vi "Field Add Test Step Fields to Table.vi"(8 "error in (no error)":errorcluster, 10 "Fields":T1[](array[typedef]), 11 "Connection Refnum":T4) -> (0 "error out":errorcluster, 3 "Connection Refnum":T4)   [LabVIEW 2011]
uses:
  SI.LIB/ODBC/SQL Controls/Connection Refnum.ctl
  Field Record.ctl
  Field DataTypes.ctl
  Field NextItem.ctl
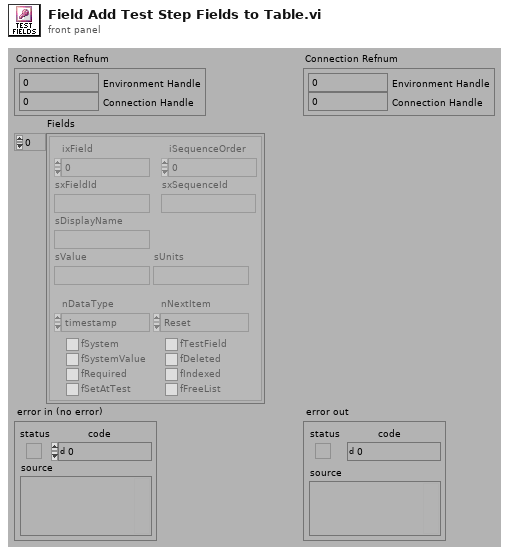
[diagram p1: front panel]
types:
  T1 = typedef "Field Record.ctl" = cluster{"ixField":i32, "iSequenceOrder":i32, "sxFieldId":string, "sxSequenceId":string, "sDisplayName":string, "sValue":string, "sUnits":string, "nDataType":T2, "nNextItem":T3, "fSystem":bool, "fSystemValue":bool, "fRequired":bool, "fSetAtTest":bool, "fTestField":bool, "fDeleted":bool, "fIndexed":bool, "fFreeList":bool}
  T2 = typedef "Field DataTypes.ctl" = enum32{"text", "numeric", "list", "timestamp", "boolean"}
  T3 = typedef "Field NextItem.ctl" = enum32{"Reset", "Retain", "Auto-Increment"}
  T4 = typedef "Connection Refnum.ctl" = cluster{"Environment Handle":i32, "Connection Handle":i32}
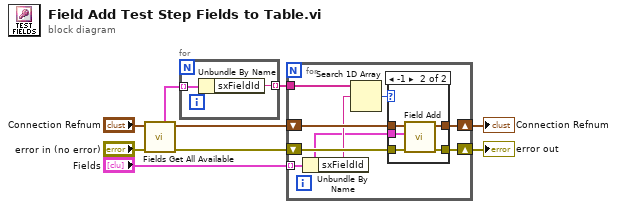
[diagram p0: block diagram]
diagram:
  n1 = call "Fields Get All Available.vi"("error in (no error)"="error in (no error)", "Connection Refnum"="Connection Refnum") -> ("error out"=w4:errorcluster, "Connection Refnum"=w5:T4, "Test Fields"=w1:T1[])  [unwired: 3 in, 4 out]
  n2 = for {
    tunnel: w1 -> [w11] mode=indexing
    tunnel: [w10] -> w2 mode=indexing
    n3 = Unbundle By Name(w11) -> ("sxFieldId"=w10:string)
  }
  n4 = for {
    shift-right: [w19] -> w8
    shift-left: w5 -> [w16]
    shift-right: [w18] -> w6
    shift-left: w4 -> [w17]
    tunnel: "Fields" -> [w12] mode=indexing
    tunnel: w2 -> [w15]
    n5 = Unbundle By Name(w12) -> ("sxFieldId"=w14:string)
    n6 = Search 1D Array(1D array=w15, element=w14) -> (index of element=w13:i32)  [unwired: 1 out]
    n7 = case shown="-1" w13 {
      tunnel: [w21 w26] -> w19
      tunnel: [w20 w25] -> w18
      tunnel: w17 -> [w20 w24]
      tunnel: w16 -> [w21 w23]
      tunnel: w12 -> [_ w22]
      frame Default {
      }
      frame -1 {
        n8 = call "Field Add.vi"("error in (no error)"=w24, "Field Record"=w22, "Connection Refnum"=w23) -> ("error out"=w25:errorcluster, "Connection Refnum"=w26:T4)  [unwired: 1 in, 6 out]
      }
    }
  }
  "Connection Refnum" <- w8
  "error out" <- w6
